vi "yellowtotedetection3.vi"(0 "Image In":T2, 2 "Minimum Score (Object Tracking 1)":i32=600, 7 "error in":errorcluster) -> (20 "Image Out":T2, 21 "Objects (pixel) (Object Tracking 1)":T1(array[cluster]), 22 "Objects (real-world) (Object Tracking 1)":T1(array[cluster]), 27 "error out":errorcluster)   [LabVIEW 2014]
uses:
  <vilib>/vision/Image Controls.llb/IMAQ Image.ctl
  <vilib>/vision/Tracking.llb/IMAQ Object Tracking SessionType.ctl
  <vilib>/vision/Vision Assistant Utils.llb/IVA Object Tracking - Init Function.ctl
  <vilib>/vision/NI_Vision_Development_Module.lvlib
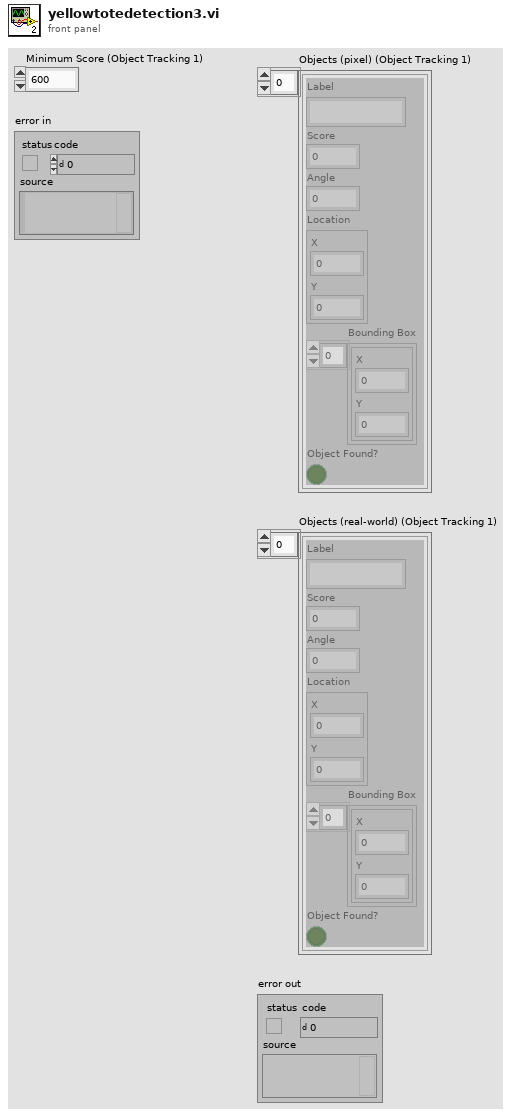
[diagram p1: front panel]
types:
  T1 = cluster{"Label":string, "Score":i32, "Angle":dbl, "Location":cluster{"X":dbl, "Y":dbl}, "Bounding Box":cluster{"X":dbl, "Y":dbl}[], "Object Found?":bool}[]
  T2 = typedef "IMAQ Image.ctl" = refnum<image>
  T3 = cluster{"Number of Histogram Bins":i32, "Blending Parameter (%)":dbl, "Max Scale Change (%)":dbl, "Max Rotation Change":dbl, "Max Shape Change (%)":dbl, "Maximum Iterations":i32}
  T4 = typedef "IVA Object Tracking - Init Function.ctl" = enum16{"Init", "Get", "Set"}
  T5 = cluster{"Initial Position":cluster{"Source":enum16{"Constant", "Measure"}, "Point ID":cluster{"GUID":string, "Index":i32}, "Point":cluster{"x":sgl, "y":sgl}}, "Initial Angle":cluster{"Source":enum16{"Constant", "Measure"}, "Measure ID":cluster{"GUID":string, "Index":i32}, "Value":dbl}}[]
  T6 = typedef "IMAQ Object Tracking SessionType.ctl" = i32
  T7 = cluster{"histogram":u32[], "Minimal Value":sgl, "Maximal Value":sgl, "Starting Value":sgl, "Interval Width":sgl, "Mean Value":sgl, "Standard  Variation":sgl, "Area (pixels)":i32}
  T8 = typedef "Image Type" = u32
  T9 = cluster{"Number of Histogram Bins":i32, "Blending Parameter (%)":dbl, "Maximum Iterations":i32}
  T10 = typedef "IMAQ Object Tracking Session.ctl" = refnum<k20>
  T11 = cluster{"Source":enum16{"Constant", "Measure"}, "Point ID":cluster{"GUID":string, "Index":i32}, "Point":cluster{"x":sgl, "y":sgl}}
  T12 = cluster{"Source":enum16{"Constant", "Measure"}, "Measure ID":cluster{"GUID":string, "Index":i32}, "Value":dbl}
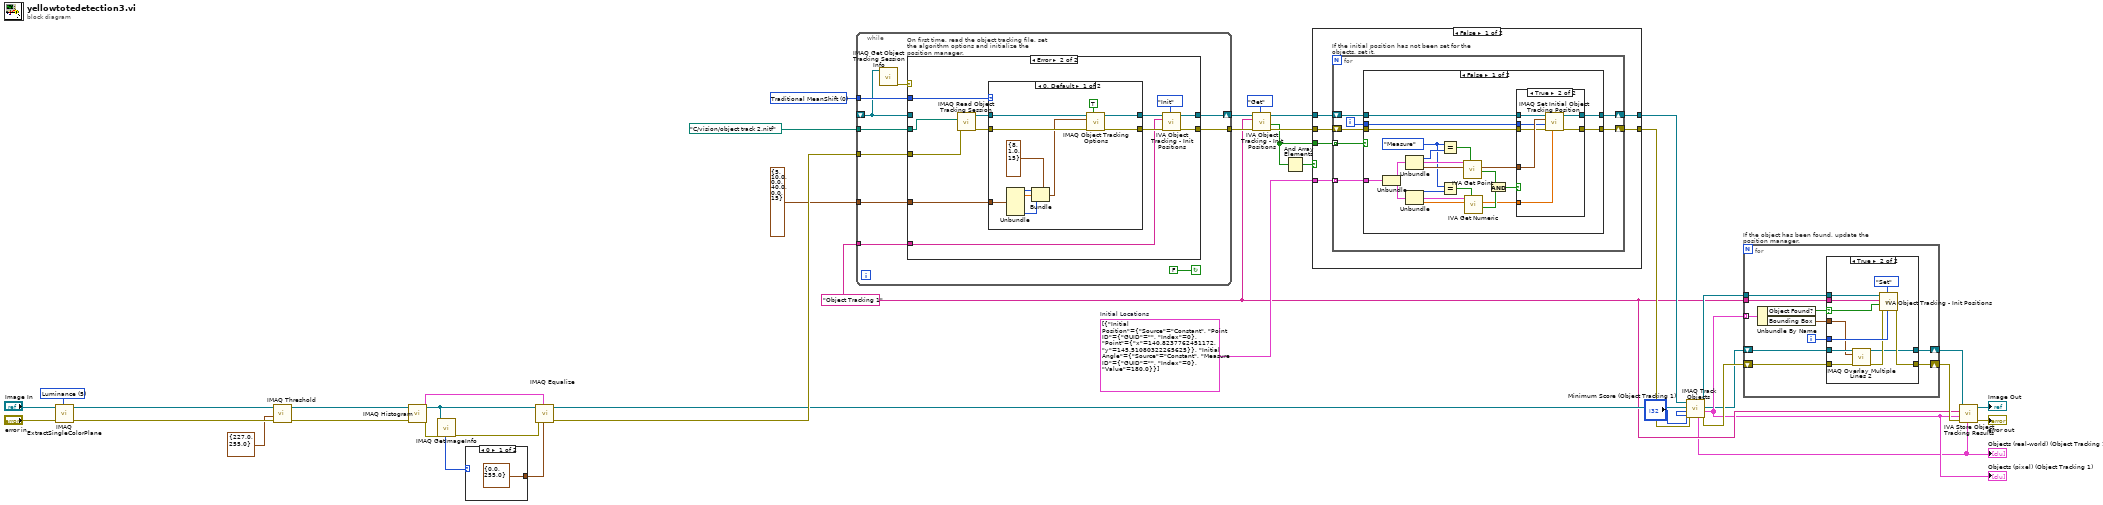
[diagram p0: block diagram]
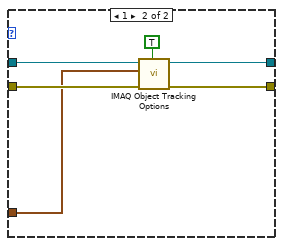
[diagram p7: hidden frame]
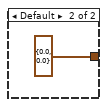
[diagram p8: hidden frame]
diagram:
  w6 = "Object Tracking 1" ("Step Name")
  w21 = T5 [{"Initial Position"={"Source"=enum."Constant", "Point ID"={"GUID"="", "Index"=0}, "Point"={"x"=140.82378, "y"=145.5108}}, "Initial Angle"={"Source"=enum."Constant", "Measure ID"={"GUID"="", "Index"=0}, "Value"=180.0}}]  # Initial Locations
  w23 = T6 0 items=["Traditional MeanShift", "Shape Adapted MeanShift"] ("Algorithm")
  w39 = 5 items=["Red", "Green", "Blue", "Hue", "Saturation", "Luminance", "Value", "Intensity"] ("Color Plane")
  n1 = call "IMAQ ExtractSingleColorPlane"("Color Plane"=w39, "error in (no error)"="error in", "Image Src"="Image In") -> ("error out"=w36:errorcluster, "Image Dst Out"=w34:T2)  [unwired: 1 in, 6 out]
  n2 = call "IMAQ Threshold"("error in (no error)"=w36, "Range"=cluster{"Lower value":sgl, "Upper value":sgl} {"Lower value"=227.0, "Upper value"=255.0}, "Image Src"=w34) -> ("error out"=w33:errorcluster, "Image Dst Out"=w29:T2)  [unwired: 3 in, 4 out]
  n3 = call "IMAQ Histogram"("error in (no error)"=w33, "Image"=w29) -> ("error out"=w28:errorcluster, "Histogram Report"=w31:T7)  [unwired: 3 in, 5 out]
  n4 = call "IMAQ GetImageInfo"("error in (no error)"=w28, "Image"=w29) -> ("error out"=w27:errorcluster, "Image Type"=w30:T8)  [unwired: 8 out]
  n5 = case shown="0" w30 {
    tunnel: [cluster{"Minimum":sgl, "Maximum":sgl} {"Minimum"=0.0, "Maximum"=255.0} ("Range") cluster{"Minimum":sgl, "Maximum":sgl} {"Minimum"=0.0, "Maximum"=0.0} ("Range")] -> w26
    frame 0 {
    }
    frame Default {
    }
  }
  n6 = call "IMAQ Equalize"("Range"=w26, "Histogram Report"=w31, "error in (no error)"=w27, "Image Src"=w29) -> ("error out"=w32:errorcluster, "Image Dst Out"=w24:T2)  [unwired: 2 in, 4 out]
  n7 = while {
    shift-right: [w51] -> w19
    shift-left: _ -> [w42]
    tunnel: path "C:/vision/object track 2.nitf" ("Tracking Session File Path") -> [w49]
    tunnel: w32 -> [w48]
    tunnel: w23 -> [w47]
    tunnel: [w46] -> w16
    tunnel: T3 {"Number of Histogram Bins"=5, "Blending Parameter (%)"=10.0, "Max Scale Change (%)"=0.0, "Max Rotation Change"=40.0, "Max Shape Change (%)"=0.0, "Maximum Iterations"=15} ("Options") -> [w45]
    tunnel: w6 -> [w44]
    stop <- FALSE continue-if-true
    n8 = call "IMAQ Get Object Tracking Session Info"("Object Tracking Session In"=w42) -> ("error out"=w43:errorcluster)  [unwired: 1 in, 9 out]
    n9 = case "On first time, read the object tracking file, set the algorithm options and initialize the position manager." shown="Error" w43 {
      tunnel: [w53 w59] -> w51
      tunnel: w42 -> [w53 _]
      tunnel: w49 -> [_ w54]
      tunnel: w48 -> [w52 w65]
      tunnel: w47 -> [_ w64]
      tunnel: [w52 w58] -> w46
      tunnel: w45 -> [_ w61]
      tunnel: w44 -> [_ w55]
      frame No Error {
      }
      frame Error {
        n10 = call "IMAQ Read Object Tracking Session"("error in (no error)"=w65, "Object Tracking Session File Path"=w54) -> ("error out"=w62:errorcluster, "Object Tracking Session Out"=w63:T10)  [unwired: 1 in, 7 out]
        n11 = case shown="0, Default" w64 {
          tunnel: w63 -> [w76 w82]
          tunnel: [w75 w81] -> w60
          tunnel: w62 -> [w74 w80]
          tunnel: [w73 w79] -> w57
          tunnel: w61 -> [w72 w78]
          frame 0, Default {
            n12 = Unbundle(w72) -> ("Number of Histogram Bins"=w71:i32, "Blending Parameter (%)"=w70:dbl, "Maximum Iterations"=w66:i32)  [unwired: 3 out]
            n13 = Bundle(cluster=T9 {"Number of Histogram Bins"=8, "Blending Parameter (%)"=1.0, "Maximum Iterations"=15} ("Mean Shift Options in"), "Number of Histogram Bins"=w71, "Blending Parameter (%)"=w70, "Maximum Iterations"=w66) -> (w69:T9)
            n14 = call-poly "IMAQ Object Tracking Options"("Get/Set (Get)"=TRUE, "error in (no error)"=w74, "Mean Shift Options in"=w69, "Object Tracking Session In"=w76) -> ("error out"=w73:errorcluster, "Object Tracking Session Out"=w75:T10)  [unwired: 1 in, 5 out]
          }
          frame 1 {
            n15 = call-poly "IMAQ Object Tracking Options"("Get/Set (Get)"=TRUE, "error in (no error)"=w80, "Shape Adapted Options in"=w78, "Object Tracking Session In"=w82) -> ("error out"=w79:errorcluster, "Object Tracking Session Out"=w81:T10)  [unwired: 2 in, 4 out]
          }
        }
        n16 = call <vilib>:"IVA Object Tracking - Init Positions.vi"("Function"=IVA_Object_Tracking_-_Init_Function."Init", "error in (no error)"=w57, "Process ID"=w55, "Object Tracking Session In"=w60) -> ("error out"=w58:errorcluster, "Object Tracking Session dup"=w59:T10)  [unwired: 2 in, 4 out]
      }
    }
  }
  n17 = call <vilib>:"IVA Object Tracking - Init Positions.vi"("Function"=IVA_Object_Tracking_-_Init_Function."Get", "error in (no error)"=w16, "Process ID"=w6, "Object Tracking Session In"=w19) -> ("error out"=w15:errorcluster, "Init Values Out"=w13:bool[], "Object Tracking Session dup"=w18:T10)  [unwired: 2 in, 3 out]
  n18 = And Array Elements(Boolean array=w13) -> (logical AND=w14:bool)
  n19 = case shown="False" w14 {
    tunnel: w21 -> [w88 _]
    tunnel: [w87 w130] -> w20
    tunnel: w18 -> [w86 w130]
    tunnel: w15 -> [w85 w129]
    tunnel: w13 -> [w84 _]
    tunnel: [w83 w129] -> w12
    frame False {
      n20 = for "If the initial position has not been set for the objects, set it." {
        tunnel: w88 -> [w94] mode=indexing
        shift-right: [w92] -> w87
        shift-left: w86 -> [w95]
        shift-right: [w89] -> w83
        shift-left: w85 -> [w91]
        tunnel: w84 -> [w90] mode=indexing
        i -> [w93]
        n21 = case shown="False" w90 {
          tunnel: w95 -> [w117 w128]
          tunnel: w94 -> [w116 _]
          tunnel: w93 -> [w100 _]
          tunnel: [w98 w128] -> w92
          tunnel: w91 -> [w97 w127]
          tunnel: [w96 w127] -> w89
          frame False {
            w106 = enum16{"Constant", "Measure"}."Measure" ("Source")
            n22 = Unbundle(w116) -> ("Initial Position"=w115:T11, "Initial Angle"=w114:T12)
            n23 = Unbundle(w115) -> ("Source"=w109:enum16{"Constant", "Measure"}, "Point ID"=w113:cluster{"GUID":string, "Index":i32}, "Point"=w112:cluster{"x":sgl, "y":sgl})
            n24 = Unbundle(w114) -> ("Source"=w107:enum16{"Constant", "Measure"}, "Measure ID"=w111:cluster{"GUID":string, "Index":i32}, "Value"=w110:dbl)
            n25 = Equal?(x=w106, y=w109) -> (x = y?=w108:bool)
            n26 = Equal?(x=w106, y=w107) -> (x = y?=w105:bool)
            n27 = call <vilib>:"IVA Get Point.vi"("Point Source"=w108, "Point in"=w112, "Point ID"=w113) -> ("Available?"=w104:bool, "Point out"=w101:cluster{"x":sgl, "y":sgl})  [unwired: 1 in, 6 out]
            n28 = call <vilib>:"IVA Get Numeric.vi"("Source"=w105, "Numeric in"=w110, "Result ID"=w111) -> ("Available?"=w103:bool, "Numeric out"=w99:dbl)  [unwired: 1 in, 6 out]
            n29 = And(x=w104, y=w103) -> (x .and. y?=w102:bool)
            n30 = case shown="True" w102 {
              tunnel: w117 -> [w119 w126]
              tunnel: w101 -> [_ w125]
              tunnel: w100 -> [_ w124]
              tunnel: w99 -> [_ w120]
              tunnel: [w119 w123] -> w98
              tunnel: w97 -> [w118 w122]
              tunnel: [w118 w121] -> w96
              frame False {
              }
              frame True {
                n31 = call "IMAQ Set Initial Object Tracking Position"("Initial Angle"=w120, "error in (no error)"=w122, "Object Index"=w124, "Position"=w125, "Object Tracking Session In"=w126) -> ("error out"=w121:errorcluster, "Object Tracking Session Out"=w123:T10)  [unwired: 5 out]
              }
            }
          }
          frame True {
          }
        }
      }
    }
    frame True {
    }
  }
  n32 = call "IMAQ Track Objects"("error in (no error)"=w12, "Minimum Score"="Minimum Score (Object Tracking 1)", "Image"=w24, "Object Tracking Session In"=w20) -> ("error out"=w11:errorcluster, "Objects (pixel)"=w5:T1, "Image (duplicate)"=w2:T2, "Object Tracking Session Out"=w10:T10, "Objects (real-world)"=w4:T1)  [unwired: 3 out]
  "Objects (pixel) (Object Tracking 1)" <- w5
  "Objects (real-world) (Object Tracking 1)" <- w4
  n33 = for "If the object has been found, update the position manager." {
    tunnel: w5 -> [w140] mode=indexing
    tunnel: w6 -> [w139]
    shift-right: [w136] -> w8
    shift-left: w11 -> [w133]
    tunnel: w10 -> [w138]
    shift-right: [w132] -> w1
    shift-left: w2 -> [w134]
    i -> [w135]
    n34 = Unbundle By Name(w140) -> ("Object Found?"=w137:bool, "Bounding Box"=w131:cluster{"X":dbl, "Y":dbl}[])
    n35 = case shown="True" w137 {
      selector: w137 -> [_ w150]
      tunnel: w139 -> [_ w152]
      tunnel: w138 -> [_ w151]
      tunnel: [w142 w149] -> w136
      tunnel: w135 -> [_ w148]
      tunnel: w134 -> [w141 w147]
      tunnel: w133 -> [w142 w145]
      tunnel: [w141 w144] -> w132
      tunnel: w131 -> [_ w143]
      frame False {
      }
      frame True {
        n36 = call "IMAQ Overlay Multiple Lines 2"("Image"=w147, "Line End Points"=w143, "error in (no error)"=w145) -> ("Image Out"=w144:T2, "error out"=w146:errorcluster)  [unwired: 11 in]
        n37 = call <vilib>:"IVA Object Tracking - Init Positions.vi"("Index"=w148, "Function"=IVA_Object_Tracking_-_Init_Function."Set", "error in (no error)"=w146, "Value"=w150, "Process ID"=w152, "Object Tracking Session In"=w151) -> ("error out"=w149:errorcluster)  [unwired: 5 out]
      }
    }
  }
  n38 = call <vilib>:"IVA Store Object Tracking Results.vi"("Objects (real-world)"=w4, "error in (no error)"=w8, "Objects (pixel)"=w5, "Step Name"=w6, "Image in"=w1) -> ("error out"=→"error out":errorcluster, "Image dup"=→"Image Out":T2)  [unwired: 5 out]
